vi "Wait on Listener.vi"(8 "error in":errorcluster, 10 "timeout ms (wait forever: -1)":i32, 11 "TCP slave in":refnum<class "TCP Server.lvclass">) -> (0 "error out":errorcluster, 1 "Timed Out":bool, 2 "connection reference":refnum<data-value>, 3 "TCP slave out":refnum<class "TCP Server.lvclass">)   [LabVIEW 2021, in "WebSockets.lvlib" / "TCP Server.lvclass"]
doc: "Wrapper for the wait on listener VI, using the listener stored in the slave and an infinite timeout. When a connection is established, the output class will contain the new connection."
uses:
  TCP Server.lvclass
  D:/my_projects/projects/Algorithms/Labview/21/WebSockets/Source/WebSockets/WebSocket/WebSocket.lvclass
  Connection.ctl
  TCP Server.lvclass/TCP Server.ctl
  WebSocket/WebSocket.lvclass/WebSocket.ctl
  Sockets/VISA TCP Socket/VISA TCP.lvclass
  D:/my_projects/projects/Algorithms/Labview/21/WebSockets/Source/Sockets/Socket/Socket.lvclass
  Sockets/VISA TCP Socket/VISA TCP.lvclass/VISA TCP.ctl
  WebSocket/WebSocket.lvclass
  D:/my_projects/projects/Algorithms/Labview/21/WebSockets/Source/WebSockets/WebSocket Server/WebSocket Server.lvclass
  D:/my_projects/projects/Algorithms/Labview/21/WebSockets/Source/WebSockets/WebSocket Server/TCP Server/TCP Server.lvclass
  D:/my_projects/projects/Algorithms/Labview/21/WebSockets/Source/Sockets/VISA TCP Socket/VISA TCP.lvclass
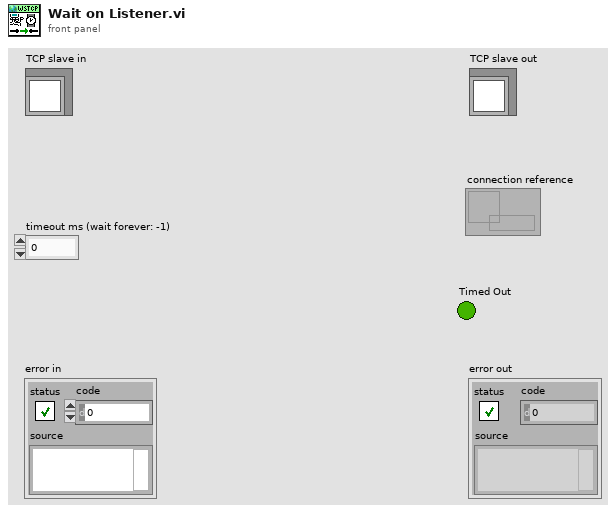
[diagram p1: front panel]
types:
  T1 = typedef "WebSockets.lvlib/TCP Server.lvclass/Connection.ctl" = cluster{"Connected?":bool, "IP address":string, "connection error":errorcluster}
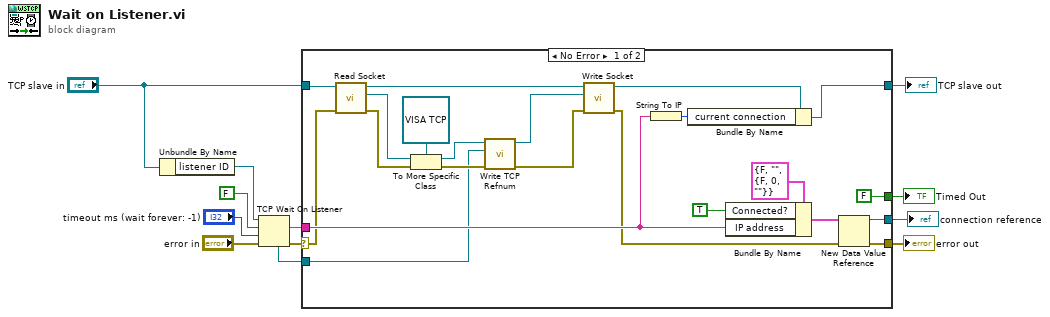
[diagram p0: block diagram]
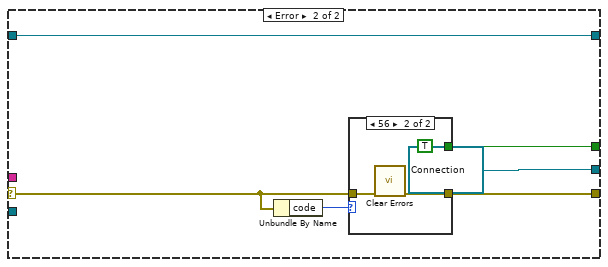
[diagram p2: hidden frame]
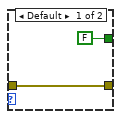
[diagram p3: hidden frame]
diagram:
  n1 = Unbundle By Name("TCP slave in") -> ("listener ID"=w10:refnum<k5>)
  n2 = TCP Wait On Listener(8:"error in", 9:"timeout ms (wait forever: -1)", 10:FALSE ("resolve remote address (T)"), 11:w10) -> (0:w5:errorcluster, 2:w1:string, 4:w9:refnum<k5>)  [unwired: 2 out]
  n3 = case shown="No Error" w5 {
    selector: w5 -> [w14 w39]
    tunnel: "TCP slave in" -> [w23 w36]
    tunnel: w9 -> [w13 _]
    tunnel: [w26 w36] -> w6
    tunnel: [w29 w38] -> w4
    tunnel: [FALSE w37] -> w3
    tunnel: [w33 refnum<data-value> refnum ("data value reference")] -> w2
    tunnel: w1 -> [w28 _]
    frame No Error {
      n4 = call "Read Socket.vi"("error in (no error)"=w14, "WebSocket in"=w23) -> ("error out"=w22:errorcluster, "Socket"=w20:refnum<class "Socket.lvclass">, "WebSocket out"=w16:refnum<class "TCP Server.lvclass">)  [unwired: 7 in]
      n5 = To More Specific Class(target class=refnum<class "VISA TCP.lvclass"> refnum ("VISA TCP out"), reference=w20, error in=w22) -> (specific class reference=w18:refnum<class "VISA TCP.lvclass">, error out=w19:errorcluster)
      n6 = call "Write TCP Refnum.vi"("error in (no error)"=w19, "TCP Refnum"=w13, "VISA TCP in"=w18) -> ("error out"=w15:errorcluster, "VISA TCP out"=w17:refnum<class "VISA TCP.lvclass">)  [unwired: 7 in]
      n7 = call "Write Socket.vi"("error in (no error)"=w15, "Socket"=w17, "WebSocket in"=w16) -> ("error out"=w24:errorcluster, "WebSocket out"=w25:refnum<class "TCP Server.lvclass">)  [unwired: 7 in]
      n8 = String To IP(1:w28) -> (0:w27:u32)
      n9 = Bundle By Name(cluster=w25, "current connection"=w27) -> (w26:refnum<class "TCP Server.lvclass">)
      n10 = Bundle By Name(cluster=T1 {"Connected?"=FALSE, "IP address"="", "connection error"={"status"=FALSE, "code"=0, "source"=""}} ("Connection"), "Connected?"=TRUE, "IP address"=w28) -> (w31:T1)
      n11 = New Data Value Reference(data value=w31, error in=w24) -> (data value reference=w33:refnum<data-value>, error out=w29:errorcluster)
    }
    frame Error {
      n12 = Unbundle By Name(w39) -> ("code"=w40:i32)
      n13 = case shown="56" w40 {
        tunnel: w39 -> [w42 w45]
        tunnel: [w42 w44] -> w38
        tunnel: [FALSE TRUE] -> w37
        frame Default {
        }
        frame 56 {
          n14 = call <vilib>:"Clear Errors.vi"("error in (no error)"=w45) -> ("error out"=w44:errorcluster)  [unwired: 5 in, 1 out]
        }
      }
    }
  }
  "error out" <- w4
  "Timed Out" <- w3
  "connection reference" <- w2
  "TCP slave out" <- w6
